vi "Read Rank.vi"(8 "error in (no error)":errorcluster, 11 "SG SC2250 Path Group in":refnum<class "SG SC2250 Path Group.lvclass">) -> (0 "error out":errorcluster, 2 "Rank":dbl, 3 "SG SC2250 Path Group out":refnum<class "SG SC2250 Path Group.lvclass">)   [LabVIEW 2023, in "RFFixtureCharact.RFPM.lvlib" / "SG SC2250 Path Group.lvclass"]
uses:
  SG SC2250 Path Group.lvclass
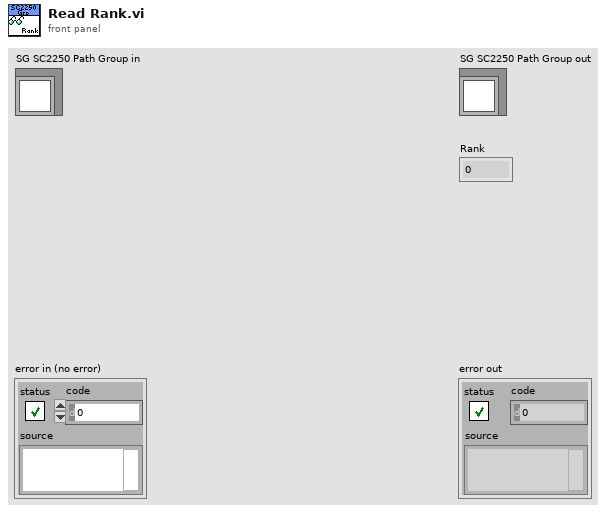
[diagram p1: front panel]
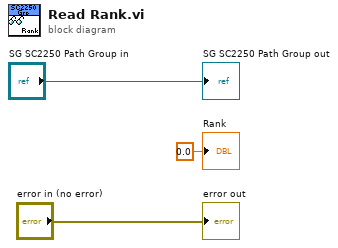
[diagram p0: block diagram]
diagram:
  "error out" <- "error in (no error)"
  "SG SC2250 Path Group out" <- "SG SC2250 Path Group in"
  "Rank" <- 0.0 ("Rank")
